vi "FpgaLink_Check_Fpga.vi"(8 "error in (no error)":errorcluster, 11 "handle":i64) -> (0 "error out":errorcluster, 2 "Is Running?":bool, 3 "handle out":i64)   [LabVIEW 2011]
doc: "Check to see if the FPGA is running.\n\nThis may only be called if flIsCommCapable() returns true. It merely verifies that the FPGA is asserting that it's ready to read. Before calling flIsFPGARunning(), you should verify that the FPGALink device actually supports CommFPGA using flIsCommCapable()."
uses:
  <vilib>/Utility/importsl/GetValueByPointer/datatype.ctl
  <vilib>/Utility/importsl/GetValueByPointer/GetValueByPointer.xnode
  libfpgalink.dll
  resource/lvimptsl.dll
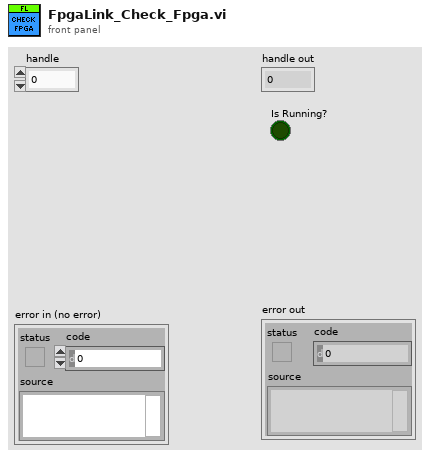
[diagram p1: front panel]
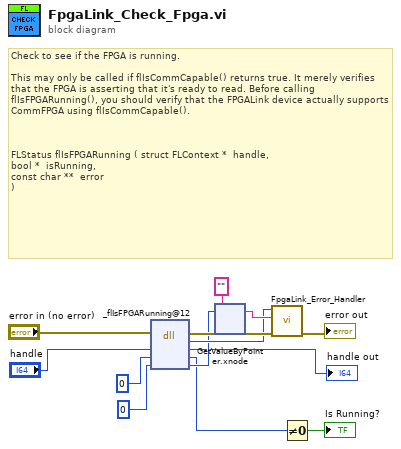
[diagram p0: block diagram]
diagram:
  # "Check to see if the FPGA is running.\n\nThis may only be called if flIsCommCapable() returns true. It merely verifies that the FPGA is asserting that it's ready to read. Before calling flIsFPGARunning(), you should verify that the FPGALink device actually supports CommFPGA using flIsCommCapable().\n\n\n\nFLStatus flIsFPGARunning\t(\tstruct FLContext * \thandle,\nbool * \tisRunning,\nconst char ** \terror \n)"
  n1 = dll-call lib="libfpgalink.*" fn="_flIsFPGARunning@12"(error in="error in (no error)", "handle"="handle", "isRunning"=u8 0, "error"=i64 0) -> (error out=w9:errorcluster, "FLStatus"=w8:u32, "handle"=→"handle out":i64, "isRunning"=w4:u8, "error"=w7:i64)  [unwired: 2 in, 1 out]
  n2 = xnode "GetValueByPointer.xnode"("Pointer"=w7, "InputType"="", "ErrorIn"=w9) -> ("Output"=w11:string, "ErrorOut"=w13:errorcluster)  [unwired: 1 in]
  n3 = call <vilib>:"FpgaLink_Error_Handler.vi"("error in (no error)"=w13, "error string"=w11, "error code"=w8) -> ("error out"=→"error out":errorcluster)  [unwired: 8 in]
  n4 = Not Equal To 0?(x=w4) -> (x != 0?=→"Is Running?":bool)
